vi "Ketihley_6221_read_data.vi"(0 "refnum":refnum<file>) -> ()   [LabVIEW 2019]
uses:
  Global/Global Variables/Data_Display_global.vi
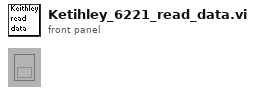
[diagram p1: front panel]
types:
  T1 = typedef "K6221_Cluster.ctl" = cluster{"Plot Window":dbl[][], "A":dbl, "A (RMS)":dbl, "Hz":dbl, "I (A)":dbl, "f (Hz)":dbl, "Update":bool, "Offset":dbl, "Offset (A)":dbl, "Compliance":bool, "Output":bool, "Output Status":bool}
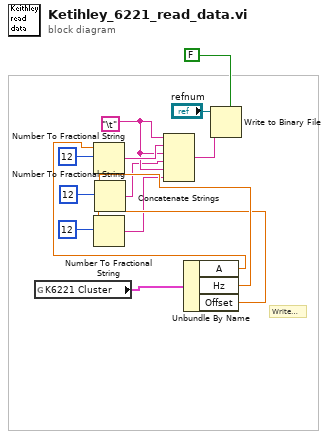
[diagram p0: block diagram]
diagram:
  w9 = "\t"
  # "Write File"
  n1 = global read "Data_Display_global.vi" "K6221 Cluster"() -> (w6:T1)
  n2 = Unbundle By Name(w6) -> ("A"=w5:dbl, "Hz"=w4:dbl, "Offset"=w3:dbl)
  n3 = Number To Fractional String(number=w5, precision (6)=i16 12) -> (F-format string=w12:string)  [unwired: 2 in]
  n4 = Number To Fractional String(number=w3, precision (6)=i16 12) -> (F-format string=w2:string)  [unwired: 2 in]
  n5 = Number To Fractional String(number=w4, precision (6)=i16 12) -> (F-format string=w1:string)  [unwired: 2 in]
  n6 = Concatenate Strings(w9, w12, w9, w1, w9, w2) -> (w13:string)
  n7 = Write to Binary File ("Write File")(file (use dialog)="refnum", data=w13, 5:FALSE ("prepend array or string size? (T)")) -> ()  [unwired: 3 in, 3 out]
